vi "DSC TSV Process Files.vi"(7 "reference":refnum<vi>, 8 "error in (no error)":errorcluster, 9 "Files":path[][](array[path]), 10 "PGSQL Paths":string[](array[string]), 11 "LV-Data.PGSQL in":refnum<class "LV-Data.PGSQL.lvclass">) -> (0 "error out":errorcluster, 3 "processed files":string[][](array[string]))   [LabVIEW 2019, in "LV-Data.PGSQL.lvclass"]
uses:
  LV-Data.PGSQL.lvclass
  <vilib>/Utility/error.llb/Clear Errors.vi
  Private/INSERT Multivalue.vi
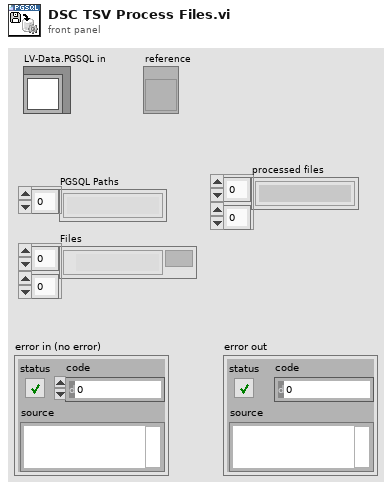
[diagram p1: front panel]
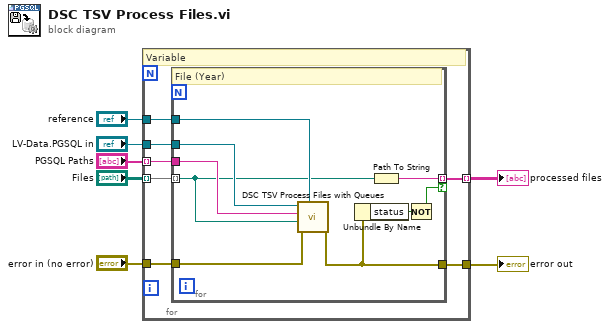
[diagram p0: block diagram]
diagram:
  n1 = for {
    tunnel: "Files" -> [w14] mode=indexing
    tunnel: "PGSQL Paths" -> [w13] mode=indexing
    tunnel: "LV-Data.PGSQL in" -> [w12]
    tunnel: "error in (no error)" -> [w11]
    tunnel: [w10] -> w1
    tunnel: [w9] -> w7 mode=indexing
    tunnel: "reference" -> [w8]
    # "Variable"
    n2 = for {
      tunnel: w14 -> [w15] mode=indexing
      tunnel: w13 -> [w16]
      tunnel: w12 -> [w17]
      tunnel: w11 -> [w19]
      tunnel: [w23] -> w10
      tunnel: [w20] -> w9 mode=indexing if=w21
      tunnel: w8 -> [w18]
      # "File (Year)"
      n3 = call "DSC TSV Process Files with Queues.vi"("reference"=w18, "error in"=w19, "File Path"=w15, "variable"=w16, "Data.PG in"=w17) -> ("error out"=w23:errorcluster)  [unwired: 6 in]
      n4 = Unbundle By Name(w23) -> ("status"=w22:bool)
      n5 = Path To String(path=w15) -> (string=w20:string)
      n6 = Not(x=w22) -> (.not. x?=w21:bool)
    }
  }
  "processed files" <- w7
  "error out" <- w1
